vi "PathCombine.vi"(10 "Path2":T2, 11 "Path1":T2) -> (3 "Combined":T2)   [LabVIEW 2014]
uses:
  TypeDefs/Point2DwSlope.ctl
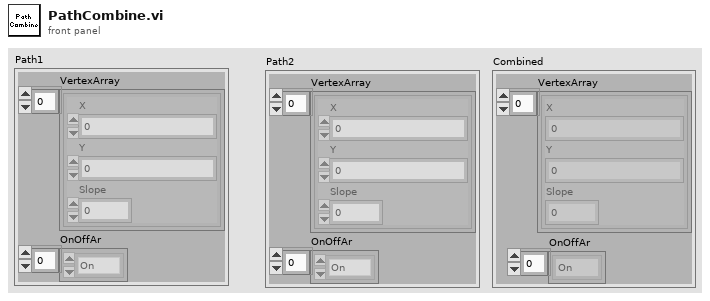
[diagram p1: front panel]
types:
  T1 = typedef "Point2DwSlope.ctl" = cluster{"X":sgl, "Y":sgl, "Slope":dbl}
  T2 = cluster{"VertexArray":T1[], "OnOffAr":enum16{"On", "Off"}[]}
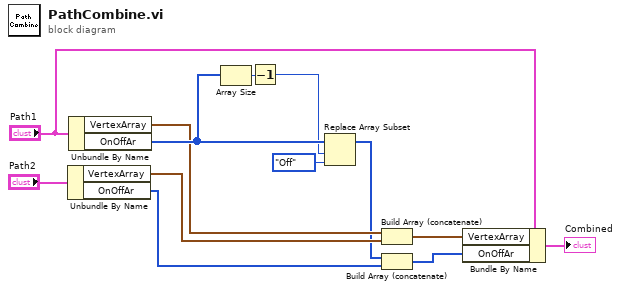
[diagram p0: block diagram]
diagram:
  n1 = Unbundle By Name("Path2") -> ("VertexArray"=w7:T1[], "OnOffAr"=w5:enum16{"On", "Off"}[])
  n2 = Unbundle By Name("Path1") -> ("VertexArray"=w8:T1[], "OnOffAr"=w12:enum16{"On", "Off"}[])
  n3 = Array Size(array=w12) -> (size(s)=w11:i32)
  n4 = Decrement(x=w11) -> (x-1=w10:i32)
  n5 = Replace Array Subset(array=w12, new element=enum16{"On", "Off"}."Off" ("new element/subarray"), index=w10) -> (w6:enum16{"On", "Off"}[])
  n6 = Build Array (concatenate)(w8, w7) -> (w3:T1[])
  n7 = Build Array (concatenate)(w6, w5) -> (w2:enum16{"On", "Off"}[])
  n8 = Bundle By Name(cluster="Path1", "VertexArray"=w3, "OnOffAr"=w2) -> (→"Combined":T2)
